vi "HIOKI PW3390 Conf Voltage.vi"(0 "VISA Resource":refnum<visa-resource-name>, 1 "Set/Query (F: Set)":bool, 2 "CH (1)":i32=1 min=1 max=4, 5 "Auto (F: OFF)":bool, 7 "Range (5: 600V)":T1(ring)=enum."600", 9 "U rect (F: RMS)":bool, 11 "error in (no error)":errorcluster, 12 "OPC query (T: ON)":bool=TRUE, 13 "Error Out (F: Off)":bool) -> (4 "VISA Resource out":refnum<visa-resource-name>, 6 "Auto out":bool, 8 "Range out":i32=600, 10 "U rect out":bool, 15 "error out":errorcluster)   [LabVIEW 2009]
doc: "Set/Query\n Set: Send the setting commands for the device.\n Query: Query the setting of the device.\n\nAuto\n Sets the voltage range to AutoRange.\n\nRange\n Sets the voltage range. Valid when the AutoRange is OFF.\n<B>Note</B>\nDepending on the measurement line combination (for 1P3W and above), the voltage range settings of other channels in the combination may be changed too.\n\nU rect\n Sets the Voltage Rectification Method to RMS/MEAN."
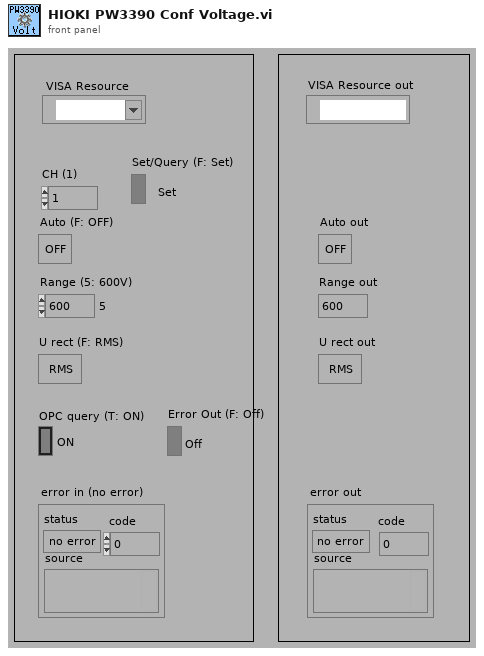
[diagram p1: front panel]
types:
  T1 = enum16{"15", "30", "60", "150", "300", "600", "1500"}
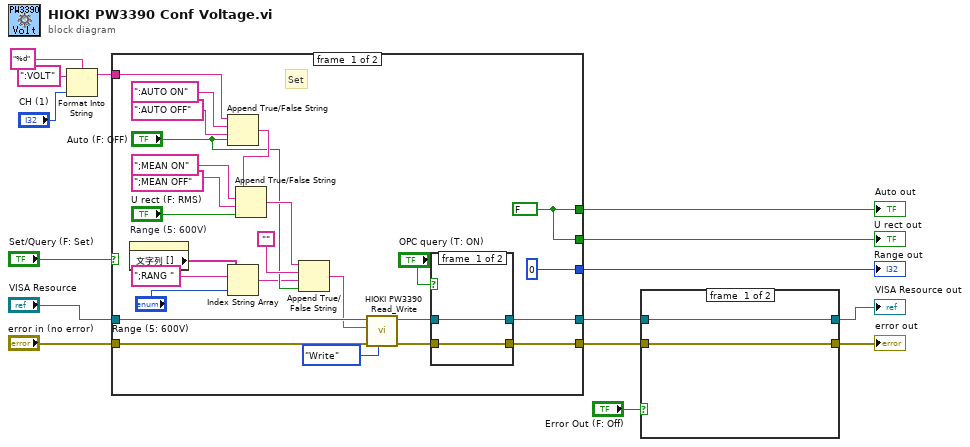
[diagram p0: block diagram]
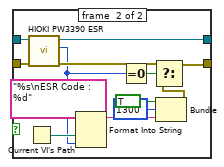
[diagram p2: hidden frame]
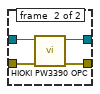
[diagram p3: hidden frame]
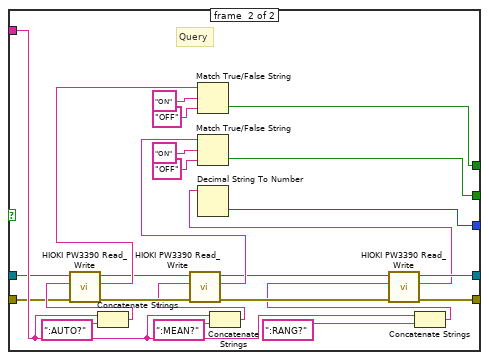
[diagram p4: hidden frame]
diagram:
  n1 = Format Into String(format string="%d", initial string=":VOLT", "CH (1)") -> (resulting string=w9:string)  [unwired: 1 in, 1 out]
  n2 = case shown="FALSE" "Set/Query (F: Set)" {
    tunnel: "error in (no error)" -> [w23 w57]
    tunnel: [w16 w50] -> w4
    tunnel: "VISA Resource" -> [w24 w60]
    tunnel: [w17 w49] -> w3
    tunnel: w9 -> [w36 w67]
    tunnel: [0 w70] -> w8
    tunnel: [w39 w64] -> w7
    tunnel: [w39 w61] -> w6
    frame #0 {
      w39 = FALSE
      # "Set"
      n3 = property on="Range (5: 600V)" class="Enum (strict)"() -> ("文字列 []"=w29:string[])  [unwired: 2 in, 2 out]
      n4 = Append True/False String(1:"Auto (F: OFF)", 2:":AUTO OFF", 3:":AUTO ON", 4:w36) -> (0:w32:string)
      n5 = Index String Array(1:"Range (5: 600V)", 2:w29, 3:";RANG ") -> (0:w25:string)
      n6 = Append True/False String(1:"U rect (F: RMS)", 2:";MEAN OFF", 3:";MEAN ON", 4:w32) -> (0:w27:string)
      n7 = Append True/False String(1:"Auto (F: OFF)", 2:w25, 3:"", 4:w27) -> (0:w22:string)
      n8 = call <instrlib>:"HIOKI PW3390 Read_Write.vi"("Read/Write"=enum16{"Read", "Write"}."Write", "error in (no error)"=w23, "data in"=w22, "VISA Resource"=w24) -> ("error out"=w18:errorcluster, "VISA Resource out"=w19:refnum<visa-resource-name>)  [unwired: 5 in, 1 out]
      n9 = case shown="TRUE" "OPC query (T: ON)" {
        tunnel: [w42 w46] -> w17
        tunnel: [w41 w45] -> w16
        tunnel: w19 -> [w42 w44]
        tunnel: w18 -> [w41 w43]
        frame #0 {
        }
        frame #1 {
          n10 = call <instrlib>:"HIOKI PW3390 OPC.vi"("error in (no error)"=w43, "VISA Resource"=w44) -> ("error out"=w45:errorcluster, "VISA Resource out"=w46:refnum<visa-resource-name>)  [unwired: 7 in, 1 out]
        }
      }
    }
    frame #1 {
      # "Query"
      n11 = Concatenate Strings(w67, ":AUTO?") -> (w58:string)
      n12 = call <instrlib>:"HIOKI PW3390 Read_Write.vi"("error in (no error)"=w57, "data in"=w58, "VISA Resource"=w60) -> ("error out"=w55:errorcluster, "data out"=w59:string, "VISA Resource out"=w56:refnum<visa-resource-name>)  [unwired: 6 in]
      n13 = Match True/False String(2:"OFF", 3:"ON", 4:w59) -> (0:w64:bool)  [unwired: 1 out]
      n14 = Concatenate Strings(w67, ":MEAN?") -> (w53:string)
      n15 = call <instrlib>:"HIOKI PW3390 Read_Write.vi"("error in (no error)"=w55, "data in"=w53, "VISA Resource"=w56) -> ("error out"=w51:errorcluster, "data out"=w54:string, "VISA Resource out"=w52:refnum<visa-resource-name>)  [unwired: 6 in]
      n16 = Match True/False String(2:"OFF", 3:"ON", 4:w54) -> (0:w61:bool)  [unwired: 1 out]
      n17 = Concatenate Strings(w67, ":RANG?") -> (w47:string)
      n18 = call <instrlib>:"HIOKI PW3390 Read_Write.vi"("error in (no error)"=w51, "data in"=w47, "VISA Resource"=w52) -> ("error out"=w50:errorcluster, "data out"=w48:string, "VISA Resource out"=w49:refnum<visa-resource-name>)  [unwired: 6 in]
      n19 = Decimal String To Number(string=w48) -> (number=w70:i32)  [unwired: 2 in, 1 out]
    }
  }
  "Auto out" <- w7
  "U rect out" <- w6
  "Range out" <- w8
  n20 = case shown="TRUE" "Error Out (F: Off)" {
    tunnel: w3 -> [w73 w86]
    tunnel: w4 -> [w72 w85]
    tunnel: [w72 w75] -> w2
    tunnel: [w73 w84] -> w1
    frame #0 {
    }
    frame #1 {
      n21 = Current VI's Path() -> (path=w82:path)
      n22 = call <instrlib>:"HIOKI PW3390 ESR.vi"("error in (no error)"=w85, "VISA Resource"=w86) -> ("error out"=w76:errorcluster, "Output Value"=w74:u8, "VISA Resource out"=w84:refnum<visa-resource-name>)  [unwired: 6 in, 1 out]
      n23 = Format Into String(format string="%s\nESR Code : %d", w82, w74) -> (resulting string=w78:string)  [unwired: 2 in, 1 out]
      n24 = Equal To 0?(x=w74) -> (x = 0?=w83:bool)
      n25 = Bundle("status"=TRUE, "code"=1300, w78) -> (w77:cluster{"status":bool, "code":i32, string})  [unwired: 1 in]
      n26 = Select(t=w76, s=w83, f=w77) -> (s? t:f=w75:errorcluster)
    }
  }
  "VISA Resource out" <- w1
  "error out" <- w2
